vi "Main.vi"() -> ()   [LabVIEW 2012]
panel:
  in  "Slide":dbl(slide) scale=0.0..10.0
  out "Waveform Chart":dbl(graph)
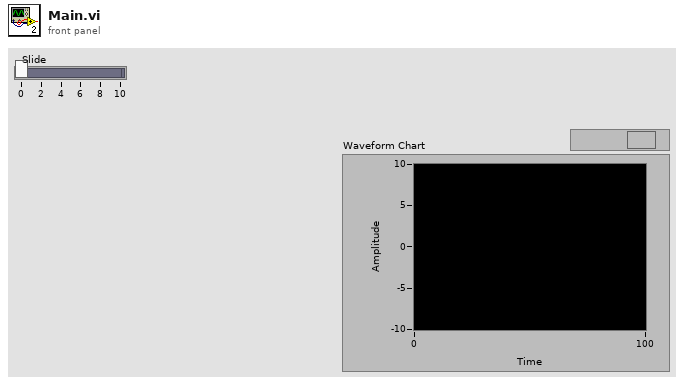
[diagram p1: front panel]
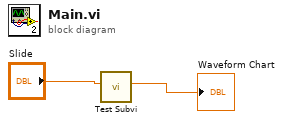
[diagram p0: block diagram]
diagram:
  n1 = call "Test Subvi.vi"("Slide"="Slide") -> ("Numeric 2"=→"Waveform Chart":dbl)  [unwired: 10 in]
